vi "font_size.vi"(10 "cell font":T1, 11 "text":string) -> (2 "height":u32, 3 "width":u32)   [LabVIEW 2017, in "rywindow.lvclass"]
uses:
  rywindow.lvclass
  <vilib>/Utility/miscctls.llb/LVFontTypeDef.ctl
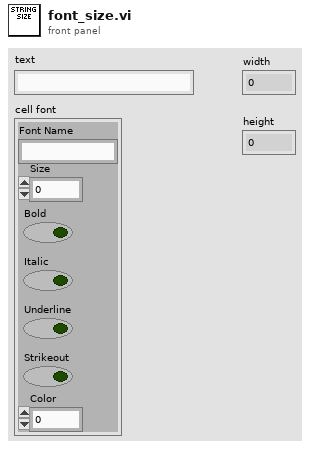
[diagram p1: front panel]
types:
  T1 = typedef "LVFontTypeDef.ctl" = cluster{"Font Name":string, "Size":u16, "Bold":bool, "Italic":bool, "Underline":bool, "Strikeout":bool, "Color":u32}
  T2 = enum16{"None", "Stacked", "Clockwise", "Counterclockwise"}
  T3 = cluster{"horizontal":enum16{"left", "center", "right"}, "vertical":enum16{"top", "center", "bottom"}}
  T4 = cluster{"Font Name:":string, "Size":i16, "Strikeout?":bool, "Italic?":bool, "Underline?":bool, "Outline?":bool, "Shadow?":bool, "Bold?":bool}
  T5 = enum16{"User-specified Font", "Application Font", "System Font", "Dialog Font"}
  T6 = cluster{"left":i16, "top":i16, "right":i16, "bottom":i16}
  T7 = cluster{"left":u32, "top":u32, "right":u32, "bottom":u32}
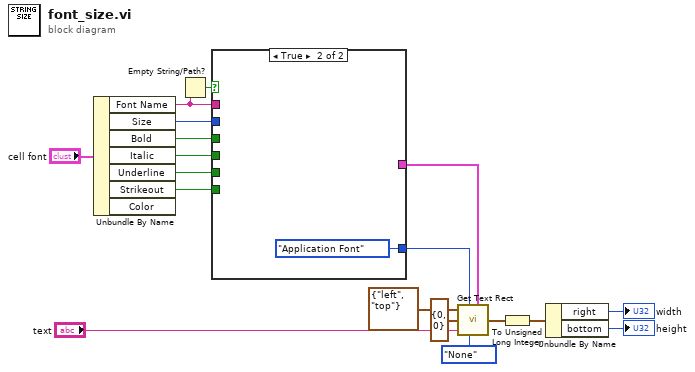
[diagram p0: block diagram]
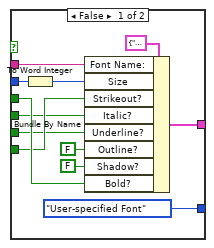
[diagram p2: hidden frame]
diagram:
  n1 = Unbundle By Name("cell font") -> ("Font Name"=w3:string, "Size"=w8:u16, "Bold"=w7:bool, "Italic"=w5:bool, "Underline"=w4:bool, "Strikeout"=w6:bool)  [unwired: 1 out]
  n2 = Empty String/Path?(string/path=w3) -> (empty?=w2:bool)
  n3 = case shown="True" w2 {
    tunnel: [T5."User-specified Font" ("desired font(Application)") T5."Application Font" ("desired font(Application)")] -> w17
    tunnel: [w28 _] -> w16
    tunnel: w3 -> [w27 _]
    tunnel: w8 -> [w26 _]
    tunnel: w7 -> [w24 _]
    tunnel: w6 -> [w23 _]
    tunnel: w5 -> [w22 _]
    tunnel: w4 -> [w21 _]
    frame False {
      n4 = To Word Integer(number=w26) -> (16bit integer=w25:i16)
      n5 = Bundle By Name(cluster=T4 {"Font Name:"="", "Size"=0, "Strikeout?"=FALSE, "Italic?"=FALSE, "Underline?"=FALSE, "Outline?"=FALSE, "Shadow?"=FALSE, "Bold?"=FALSE} ("[user-specified font]"), "Font Name:"=w27, "Size"=w25, "Strikeout?"=w23, "Italic?"=w22, "Underline?"=w21, "Outline?"=FALSE, "Shadow?"=FALSE, "Bold?"=w24) -> (w28:T4)
    }
    frame True {
    }
  }
  n6 = call <vilib>:"Get Text Rect.vi"("alignment(left, top)"=T3 {"horizontal"=enum."left", "vertical"=enum."top"}, "desired font(Application)"=w17, "origin(0,0)"=cluster{"horizontal":i16, "vertical":i16} {"horizontal"=0, "vertical"=0}, "text"="text", "text orientation"=T2."None", "[user-specified font]"=w16) -> ("rect"=w15:T6)  [unwired: 3 in]
  n7 = To Unsigned Long Integer(number=w15) -> (unsigned 32bit integer=w1:T7)
  n8 = Unbundle By Name(w1) -> ("right"=→"width":u32, "bottom"=→"height":u32)
